vi "AgilentTest.vi"() -> ()   [LabVIEW 2009]
uses:
  AgilentControl.ctl
  Channel Config.ctl
  <instrlib>/Agilent 6000 Series/Agilent 6000 Series.lvlib
panel:
  in  "Agilent Download":bool=TRUE
  out "Data Download Error":errorcluster
  out "Agilent Control Out":T1={"Trig?"=TRUE, "VISA session"="MRT_Scintillator_Scope", "Setup to Load"="4", "Timeout (ms)"=10000, "Desired Samp"=enum."100", "Captured Samp"=10, "Desired Channels"=[]}
  in  "Agilent Control In":T1={"Trig?"=FALSE, "VISA session"="MRT_Scintillator_Scope", "Setup to Load"="4", "Timeout (ms)"=10000, "Desired Samp"=enum."100", "Captured Samp"=10, "Desired Channels"=[]}
  in  "Target File Path":path=path "C:/Temp/ScintillatorScope.csv"
  out "Waveform Graph":waveform(dbl)[](graph)=[{"t0"=timestamp(-2.0200000000025753e-05 s since 1904-01-01), "dt"=1e-09, "Y"=array[200000 elements]}, {"t0"=timestamp(-2.0200000000025753e-05 s since 1904-01-01), "dt"=1e-09, "Y"=array[200000 elements]}]
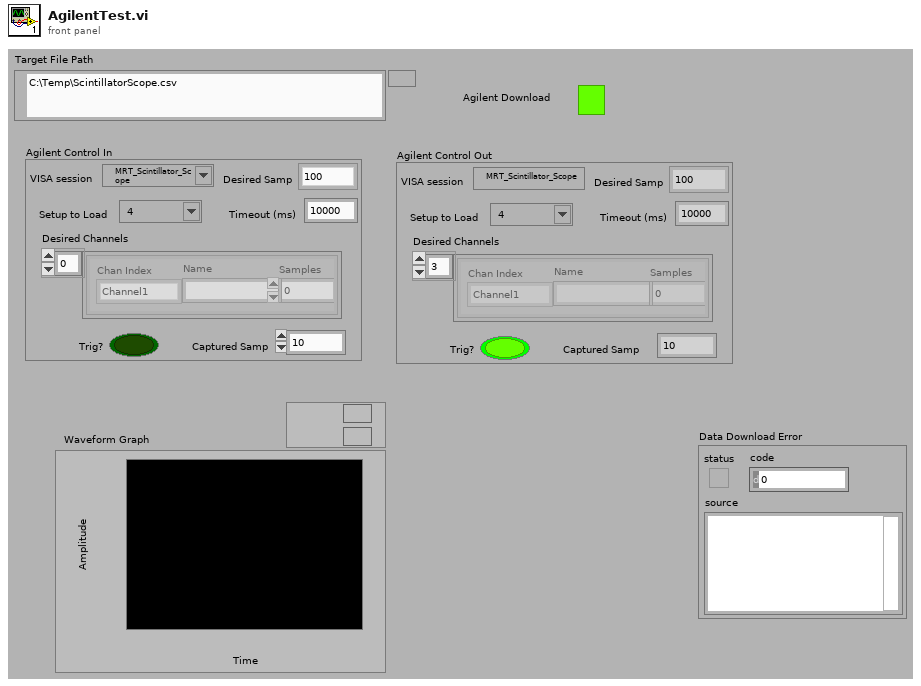
[diagram p1: front panel]
types:
  T1 = typedef "AgilentControl.ctl" = cluster{"Trig?":bool, "VISA session":refnum<visa-resource-name>, "Setup to Load":string, "Timeout (ms)":u32, "Desired Samp":enum32{"100", "250", "500", "1000", "2000", "5000", "10000", "20000", "50000", "100000", "200000", "500000", "1000000", "2000000", "4000000", "8000000"}, "Captured Samp":i32, "Desired Channels":T2[]}
  T2 = typedef "Channel Config.ctl" = cluster{"Chan Index":enum16{"Channel1", "Channel2", "Channel3", "Channel4", "MATH"}, "Name":string, "Samples":i32}
  T3 = enum32{"100", "250", "500", "1000", "2000", "5000", "10000", "20000", "50000", "100000", "200000", "500000", "1000000", "2000000", "4000000", "8000000"}
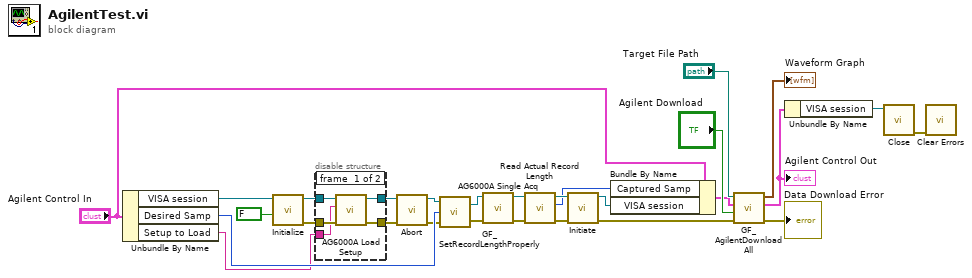
[diagram p0: block diagram]
diagram:
  n1 = Unbundle By Name("Agilent Control In") -> ("VISA session"=w14:refnum<visa-resource-name>, "Desired Samp"=w13:T3, "Setup to Load"=w12:string)
  n2 = call <instrlib>:"Initialize.vi"("Reset? (T: Yes)"=FALSE, "VISA resource name"=w14) -> ("error out"=w22:errorcluster, "VISA resource name out"=w23:refnum<visa-resource-name>)  [unwired: 8 in]
  n3 = disable-structure shown="Enabled" {
    disable-tunnel: [w33 w34] -> w7
    disable-tunnel: [w32 w35] -> w10
    disable-tunnel: w23 -> [w31 w34]
    disable-tunnel: w22 -> [w30 w35]
    disable-tunnel: w12 -> [w29 _]
    frame #0 {
      n4 = call "AG6000A Load Setup.vi"("error in (no error)"=w30, "Setup to Load"=w29, "VISA session"=w31) -> ("error out"=w32:errorcluster, "dup VISA session"=w33:refnum<visa-resource-name>)  [unwired: 7 in]
    }
    frame #1 {
    }
  }
  n5 = call <instrlib>:"Abort.vi"("error in (no error)"=w10, "VISA resource name"=w7) -> ("error out"=w9:errorcluster, "VISA resource name out"=w8:refnum<visa-resource-name>)  [unwired: 8 in]
  n6 = call "GF_SetRecordLengthProperly.vi"("error in (no error)"=w9, "Num Samples"=w13, "VISA resource name"=w8) -> ("error out"=w16:errorcluster, "VISA resource name out"=w17:refnum<visa-resource-name>)
  n7 = call "AG6000A Single Acq.vi"("error in (no error)"=w16, "VISA session"=w17) -> ("error out"=w18:errorcluster, "dup VISA session"=w19:refnum<visa-resource-name>)  [unwired: 8 in]
  n8 = call <instrlib>:"Read Actual Record Length.vi"("error in (no error)"=w18, "VISA resource name"=w19) -> ("error out"=w20:errorcluster, "Actual Record Length"=w11:i32, "VISA resource name out"=w21:refnum<visa-resource-name>)  [unwired: 7 in]
  n9 = call <instrlib>:"Initiate.vi"("error in (no error)"=w20, "VISA resource name"=w21) -> ("error out"=w4:errorcluster, "VISA resource name out"=w5:refnum<visa-resource-name>)  [unwired: 8 in]
  n10 = Bundle By Name(cluster="Agilent Control In", "Captured Samp"=w11, "VISA session"=w5) -> (w3:T1)
  n11 = call "GF_AgilentDownloadAll.vi"("Error In"=w4, "Agilent Download"="Agilent Download", "Agilent Cluster In"=w3, "File Path"="Target File Path") -> ("error out"=→"Data Download Error":errorcluster, "Agilent Cluster Out"=w2:T1, "Agilent Scintillator Scope Graph"=→"Waveform Graph":waveform(dbl)[])  [unwired: 1 in]
  "Agilent Control Out" <- w2
  n12 = Unbundle By Name(w2) -> ("VISA session"=w1:refnum<visa-resource-name>)
  n13 = call <instrlib>:"Close.vi"("VISA resource name"=w1) -> ("error out"=w28:errorcluster)  [unwired: 10 in]
  n14 = call <vilib>:"Clear Errors.vi"("error in (no error)"=w28) -> ()  [unwired: 6 in, 1 out]
